vi "Process CAN Data.vi"(4 "XNET Frames":refnum<queue>, 5 "Host Parameters":T1, 6 "Log":bool, 7 "Init?":bool, 8 "error in (no error)":errorcluster, 9 "Data Timed Out?":bool, 11 "Data":T5[](array[typedef]) {"payload" format="%x"; "timestamp" format="%<%.7X\n%x>T"; "type" items=["CAN Data"=0, "CAN Remote"=1, "CAN Bus Error"=2, "CAN 2.0 Data"=8, "CAN FD Data"=16, "CAN FD+BRS Data"=24, "J1939 Data"=192, "Delay"=224, "Log Trigger"=225, "Start Trigger"=226]; "identifier" format="%x"}) -> (0 "error out":errorcluster, 2 "Table Update":bool, 3 "Table":string[][](array[string]))   [LabVIEW 2019, in "CAN Stream Support Workspace Shared.lvlib"]
uses:
  CAN Stream Support Workspace Shared.lvlib
  <vilib>/xnet/xnet.llb/XNET Frame CAN.ctl
  <vilib>/xnet/xnet.llb/XNET Frame Type CAN.ctl
  Types/Host Stream Engine Parameters.ctl
  Addon/Addon Shared/Types/Filter Parameters.ctl
  Addon/Addon Shared/Types/Direction Filter.ctl
  Addon/Addon Shared/Types/Type Filter.ctl
  <vilib>/dlg_ctls.llb/Space Constant.vi
  <vilib>/Utility/error.llb/Trim Whitespace.vi
  Convert Time to UTC String.vi
  <vilib>/Utility/error.llb/Trim Whitespace One-Sided.vi
  <userlib>/_OpenG.lib/array/array.llb/Sort 2D Array (String)__ogtk.vi
  <userlib>/_OpenG.lib/array/array.llb/openg_array.lvlib
  Addon/Addon Shared/CAN Stream Support Shared.lvlib
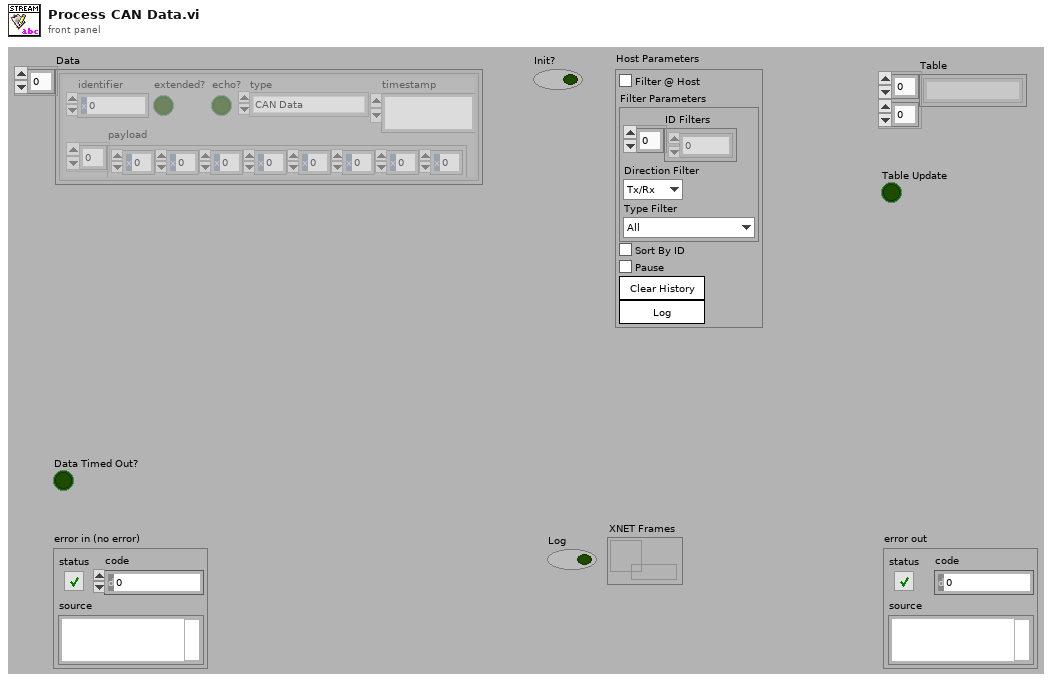
[diagram p1: front panel]
types:
  T1 = typedef "CAN Stream Support Workspace Shared.lvlib/Host Stream Engine Parameters.ctl" = cluster{"Host Filter":bool, "Filter Parameters":T2, "Sort By ID":bool, "Pause":bool, "Clear History":bool, "Log":bool}
  T2 = typedef "CAN Stream Support Shared.lvlib/Filter Parameters.ctl" = cluster{"ID Filters":u32[], "Direction Filter":T3, "Type Filter":T4}
  T3 = typedef "CAN Stream Support Shared.lvlib/Direction Filter.ctl" = enum16{"Tx/Rx", "Rx", "Tx"}
  T4 = typedef "CAN Stream Support Shared.lvlib/Type Filter.ctl" = enum16{"All", "CAN Data", "CAN Remote", "CAN Bus Error", "CAN 2.0 Data", "CAN FD Data", "CAN FD+BRS Data", "J1939 Data", "Delay", "Log Trigger", "Start Trigger"}
  T5 = typedef "XNET Frame CAN.ctl" = cluster{"timestamp":timestamp, "payload":u8[], "identifier":u32, "type":T6, "extended?":bool, "echo?":bool}
  T6 = typedef "XNET Frame Type CAN.ctl" = u8
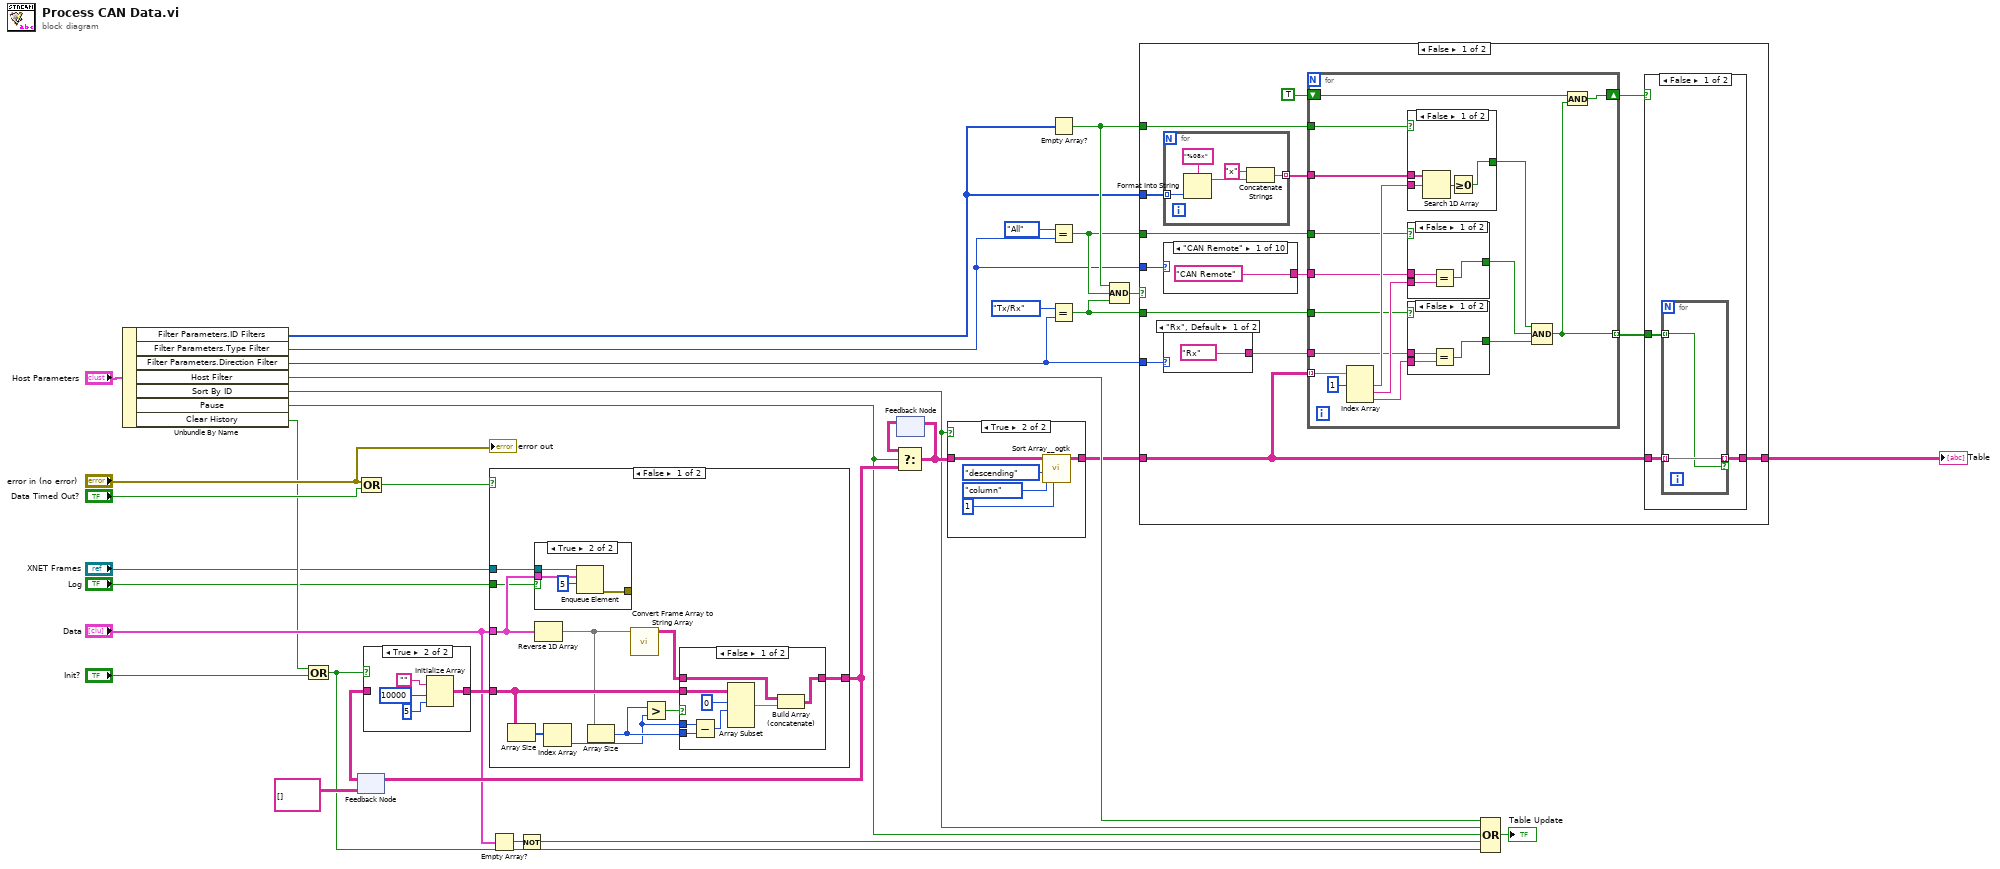
[diagram p0: block diagram]
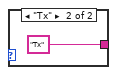
[diagram p5: hidden frame]
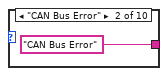
[diagram p6: hidden frame]
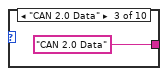
[diagram p7: hidden frame]
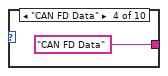
[diagram p8: hidden frame]
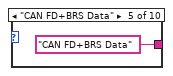
[diagram p9: hidden frame]
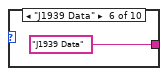
[diagram p10: hidden frame]
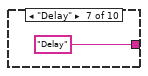
[diagram p11: hidden frame]
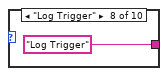
[diagram p12: hidden frame]
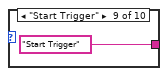
[diagram p13: hidden frame]
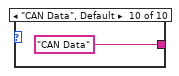
[diagram p14: hidden frame]
diagram:
  n1 = Unbundle By Name("Host Parameters") -> ("Filter Parameters.ID Filters"=w5:u32[], "Filter Parameters.Type Filter"=w4:T4, "Filter Parameters.Direction Filter"=w3:T3, "Host Filter"=w19:bool, "Sort By ID"=w15:bool, "Pause"=w14:bool, "Clear History"=w18:bool)
  n2 = Compound Arithmetic op=OR(w18, "Init?") -> (w16:bool)
  n3 = feedback #1(string[][] [] ("Sorted Array out")) -> (w32:string[][])
  n4 = Compound Arithmetic op=OR("error in (no error)", "Data Timed Out?") -> (w26:bool)
  n5 = case shown="True" w16 {
    tunnel: [w34 w36] -> w33
    tunnel: w32 -> [w34 _]
    frame False {
    }
    frame True {
      n6 = Initialize Array("", 10000 ("dimension size"), 5 ("Dimension Size")) -> (w36:string[][])
    }
  }
  n7 = case shown="False" w26 {
    tunnel: "Data" -> [w41 _]
    tunnel: w33 -> [w45 w63]
    tunnel: [w46 w63] -> w30
    tunnel: "Log" -> [w40 _]
    tunnel: "XNET Frames" -> [w39 _]
    frame False {
      n8 = Array Size(array=w45) -> (size(s)=w44:i32[])
      n9 = case shown="True" w40 {
        tunnel: w41 -> [_ w53]
        tunnel: [_ w52] -> _
        tunnel: w39 -> [_ w51]
        frame False {
        }
        frame True {
          n10 = Enqueue Element(queue=w51, element=w53, timeout in ms (-1)=5) -> (error out=w52:errorcluster)  [unwired: 1 in, 2 out]
        }
      }
      n11 = Reverse 1D Array(array=w41) -> (reversed array=w42:T5[])
      n12 = Index Array(array=w44) -> (element=w43:i32)  [unwired: 1 in]
      n13 = Array Size(array=w42) -> (size(s)=w47:i32)
      n14 = call "Convert Frame Array to String Array.vi"("Array in"=w42) -> ("Array out"=w48:string[][])  [unwired: 10 in]
      n15 = Greater?(x=w47, y=w43) -> (0:w49:bool)
      n16 = case shown="False" w49 {
        tunnel: w48 -> [w55 w62]
        tunnel: w43 -> [w61 _]
        tunnel: [w54 w62] -> w46
        tunnel: w45 -> [w59 _]
        tunnel: w47 -> [w60 _]
        frame False {
          n17 = Subtract(x=w61, y=w60) -> (x-y=w57:i32)
          n18 = Array Subset(array=w59, index (row)=0 ("index"), length (row)=w57) -> (w56:string[][])  [unwired: 2 in]
          n19 = Build Array (concatenate)(w55, w56) -> (w54:string[][])
        }
        frame True {
        }
      }
    }
    frame True {
    }
  }
  n20 = feedback-in #1(w30) -> ()
  n21 = Empty Array?(array="Data") -> (empty?=w24:bool)
  n22 = Not(x=w24) -> (.not. x?=w22:bool)
  n23 = feedback #2() -> (w29:string[][])  [unwired: 1 in]
  n24 = Select(t=w29, s=w14, f=w30) -> (s? t:f=w25:string[][])
  n25 = feedback-in #2(w25) -> ()
  n26 = case shown="True" w15 {
    tunnel: w25 -> [w64 w69]
    tunnel: [w64 w68] -> w13
    frame False {
    }
    frame True {
      n27 = call-poly <userlib>:"Sort Array__ogtk.vi"("Column/Row to Sort By"=u32 1, "Sort By in"=enum16{"row", "column"}."column", "Order"=enum16{"ascending", "descending"}."descending", "Array in"=w69) -> ("Sorted Array out"=w68:string[][])  [unwired: 4 in, 3 out]
    }
  }
  n28 = Empty Array?(array=w5) -> (empty?=w8:bool)
  n29 = Equal?(x=Type_Filter."All", y=w4) -> (x = y?=w6:bool)
  n30 = Equal?(x=Direction_Filter."Tx/Rx", y=w3) -> (x = y?=w7:bool)
  n31 = Compound Arithmetic op=AND(w8, w6, w7) -> (w10:bool)
  n32 = case shown="False" w10 {
    tunnel: w13 -> [w77 w137]
    tunnel: w6 -> [w83 _]
    tunnel: w7 -> [w82 _]
    tunnel: [w76 w137] -> w9
    tunnel: w8 -> [w81 _]
    tunnel: w5 -> [w75 _]
    tunnel: w4 -> [w73 _]
    tunnel: w3 -> [w71 _]
    frame False {
      n33 = for {
        tunnel: w75 -> [w97] mode=indexing
        tunnel: [w96] -> w74 mode=indexing
        n34 = Format Into String(format string="%08x", w97) -> (resulting string=w99:string)  [unwired: 2 in, 1 out]
        n35 = Concatenate Strings("x" ("string"), w99) -> (w96:string)
      }
      n36 = case shown="\"CAN Remote\"" w73 {
        tunnel: ["CAN Remote" "CAN Bus Error" "CAN 2.0 Data" "CAN FD Data" "CAN FD+BRS Data" "J1939 Data" "Delay" "Log Trigger" "Start Trigger" "CAN Data"] -> w72
        frame "CAN Remote" {
        }
        frame "CAN Bus Error" {
        }
        frame "CAN 2.0 Data" {
        }
        frame "CAN FD Data" {
        }
        frame "CAN FD+BRS Data" {
        }
        frame "J1939 Data" {
        }
        frame "Delay" {
        }
        frame "Log Trigger" {
        }
        frame "Start Trigger" {
        }
        frame "CAN Data", Default {
        }
      }
      n37 = case shown="\"Rx\", Default" w71 {
        tunnel: ["Rx" "Tx"] -> w70
        frame "Rx", Default {
        }
        frame "Tx" {
        }
      }
      n38 = for {
        tunnel: w77 -> [w121] mode=indexing
        tunnel: w83 -> [w108]
        tunnel: w72 -> [w109]
        tunnel: w70 -> [w110]
        tunnel: w82 -> [w111]
        tunnel: w74 -> [w122]
        tunnel: w81 -> [w123]
        tunnel: [w114] -> w79 mode=indexing
        shift-right: [w113] -> w78
        shift-left: TRUE -> [w115]
        n39 = Index Array(array=w121, index #1=1 ("index")) -> (element #1=w120:string, element #2=w119:string, element #3=w107:string)  [unwired: 2 in]
        n40 = case shown="False" w123 {
          selector: w123 -> [_ w128]
          tunnel: w122 -> [w127 _]
          tunnel: w120 -> [w126 _]
          tunnel: [w124 w128] -> w118
          frame False {
            n41 = Search 1D Array(1D array=w127, element=w126) -> (index of element=w125:i32)  [unwired: 1 in]
            n42 = Greater Or Equal To 0?(x=w125) -> (x >= 0?=w124:bool)
          }
          frame True {
          }
        }
        n43 = case shown="False" w108 {
          selector: w108 -> [_ w132]
          tunnel: w109 -> [w131 _]
          tunnel: [w130 w132] -> w117
          tunnel: w119 -> [w129 _]
          frame False {
            n44 = Equal?(x=w131, y=w129) -> (x = y?=w130:bool)
          }
          frame True {
          }
        }
        n45 = case shown="False" w111 {
          selector: w111 -> [_ w136]
          tunnel: w110 -> [w135 _]
          tunnel: [w134 w136] -> w116
          tunnel: w107 -> [w133 _]
          frame False {
            n46 = Equal?(x=w135, y=w133) -> (x = y?=w134:bool)
          }
          frame True {
          }
        }
        n47 = Compound Arithmetic op=AND(w118, w117, w116) -> (w114:bool)
        n48 = Compound Arithmetic op=AND(w115, w114) -> (w113:bool)
      }
      n49 = case shown="False" w78 {
        tunnel: w77 -> [w101 w106]
        tunnel: [w102 w106] -> w76
        tunnel: w79 -> [w103 _]
        frame False {
          n50 = for {
            tunnel: w103 -> [w104] mode=indexing
            tunnel: [w105] -> w102 mode=indexing if=w104
            tunnel: w101 -> [w105] mode=indexing
          }
        }
        frame True {
        }
      }
    }
    frame True {
    }
  }
  "Table" <- w9
  n51 = Compound Arithmetic op=OR(w19, w15, w14, w22, w16) -> (→"Table Update":bool)
  "error out" <- "error in (no error)"
